vi "Solve2.vi"(8 "Error In":errorcluster, 11 "object in":refnum<class "2021_8.lvclass">) -> (0 "Error Out":errorcluster, 2 "Result":u64, 3 "object out":refnum<class "2021_8.lvclass">)   [LabVIEW 2020, in "2021_8.lvclass"]
uses:
  2021_8.lvclass
  2021_8.lvclass/2021_8.ctl
panel:
  out "Array":i32[](array[numeric])
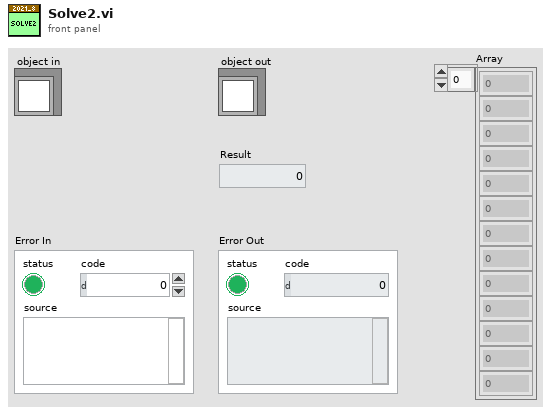
[diagram p1: front panel]
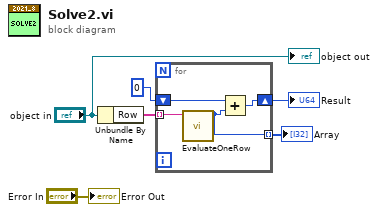
[diagram p0: block diagram]
diagram:
  n1 = Unbundle By Name("object in") -> ("Row"=w4:string[])
  n2 = for {
    tunnel: w4 -> [w10] mode=indexing
    shift-right: [w8] -> w2
    shift-left: u32 0 -> [w9]
    tunnel: [w7] -> w1 mode=indexing
    n3 = call "EvaluateOneRow.vi"("OneString"=w10) -> ("number"=w7:i32)  [unwired: 9 in, 1 out]
    n4 = Add(x=w9, y=w7) -> (x+y=w8:u32)
  }
  "Result" <- w2
  "Array" <- w1
  "Error Out" <- "Error In"
  "object out" <- "object in"
